vi "2025_day7.vi"() -> ()   [LabVIEW 2025]
uses:
  <userlib>/_OpenG.lib/string/string.llb/openg_string.lvlib
panel:
  out "Task 2":i64
  out "Task 1":i32
  in  "Switch":bool caption="Ex. Data  vs.  User Data"
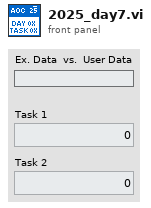
[diagram p1: front panel]
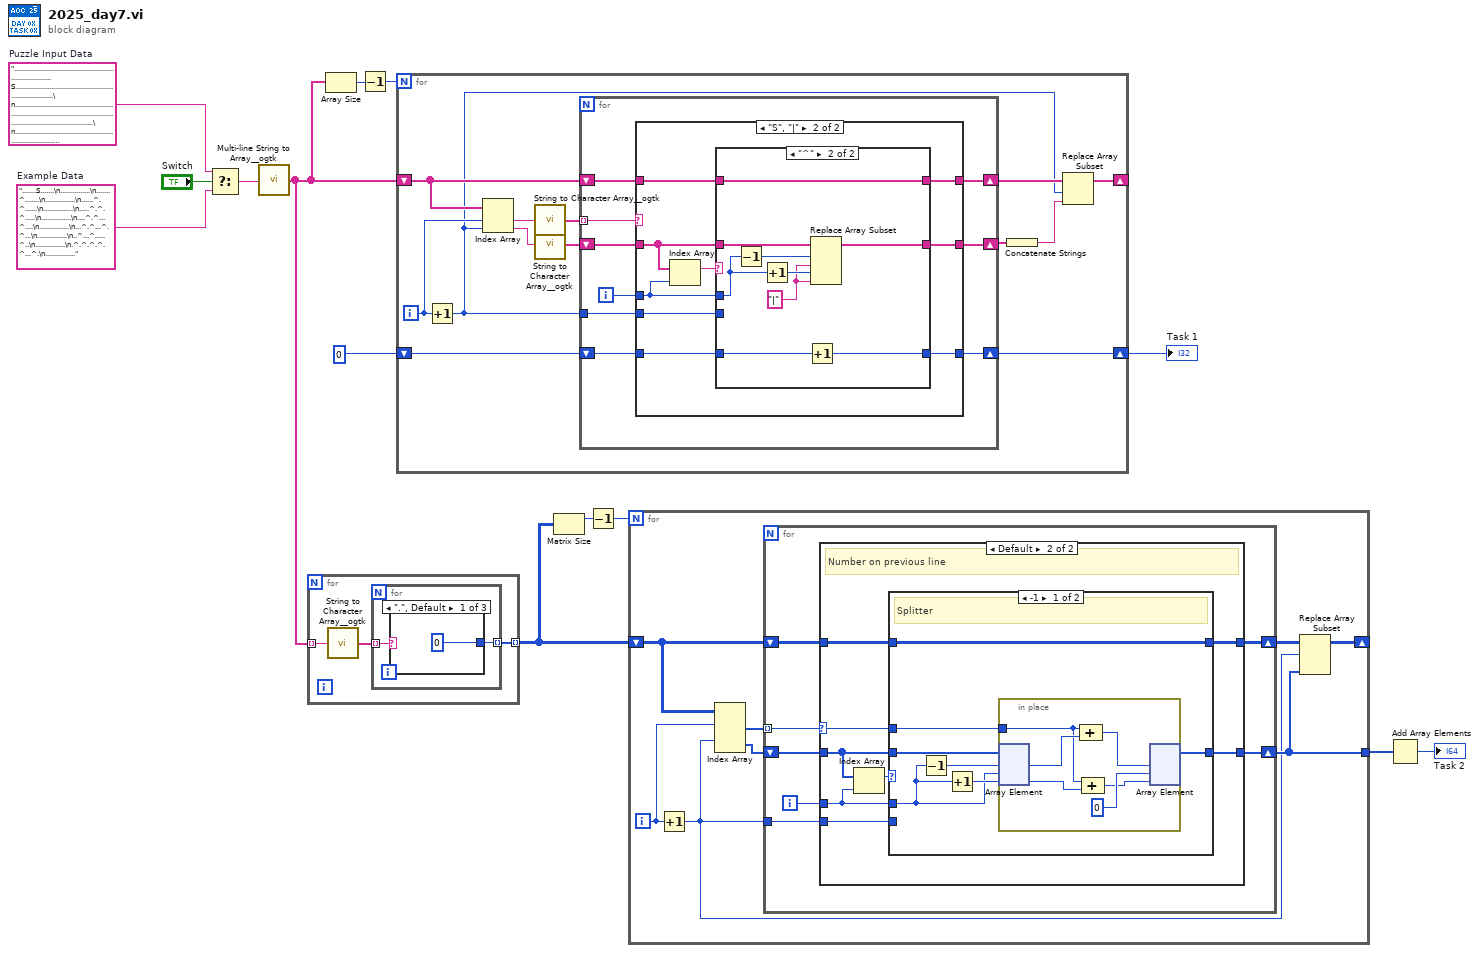
[diagram p0: block diagram]
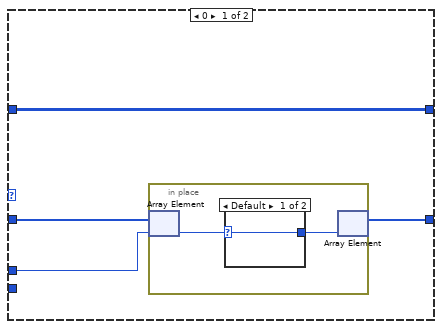
[diagram p2: hidden frame]
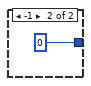
[diagram p3: hidden frame]
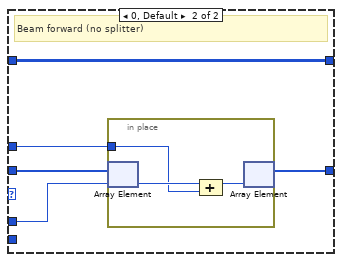
[diagram p4: hidden frame]
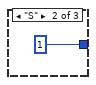
[diagram p5: hidden frame]
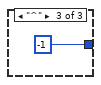
[diagram p6: hidden frame]
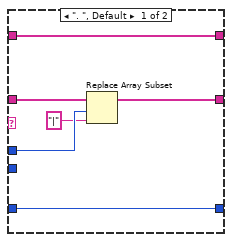
[diagram p8: hidden frame]
diagram:
  w12 = "......................................................................S......................................................................\n.............................................................................................................................................\n......................................................................^......................................................................\n.............................................................................................................................................\n.....................................................................^.^.....................................................................\n.............................................................................................................................................\n....................................................................^.^.^....................................................................\n.............................................................................................................................................\n...................................................................^.^.^.^...................................................................\n.............................................................................................................................................\n..................................................................^.^.^...^..................................................................\n.............................................................................................................................................\n.................................................................^.^.^.^.^.^.................................................................\n.............................................................................................................................................\n................................................................^.....^.^.^.^................................................................\n.............................................................................................................................................\n...............................................................^...^.^...^.^.^...............................................................\n.............................................................................................................................................\n..............................................................^.^.^.^...^.^.^.^..............................................................\n.............................................................................................................................................\n.............................................................^.^.^.^.^.^.^.^.^.^.............................................................\n.............................................................................................................................................\n............................................................^.^.^.^.^.^...^.^...^............................................................\n.............................................................................................................................................\n...........................................................^.^.^.^...^.^.^...^.^.^...........................................................\n.............................................................................................................................................\n..........................................................^.^.^...^.^.^.....^.^.^.^..........................................................\n.............................................................................................................................................\n.........................................................^.^...^...^.^.^.^...^.....^.........................................................\n.............................................................................................................................................\n........................................................^.....^.^.^...^.^.^.^.^.^.^.^........................................................\n.............................................................................................................................................\n.......................................................^.^...^.....^.......^.^.^.^...^.......................................................\n.............................................................................................................................................\n......................................................^.....^...^.^.^.^...^...^.^...^.^......................................................\n.............................................................................................................................................\n.....................................................^.^.^.^.^.^.^.^.^.....^.^.^.^...^.^.....................................................\n.............................................................................................................................................\n....................................................^.^.^.^...^.^...^.^.^...^...^.^.^.^.^....................................................\n.............................................................................................................................................\n...................................................^.....^.^.....^.^.^.^.....^.^.^.^.^.^.^...................................................\n.............................................................................................................................................\n..................................................^.^.^.^.^.^.^.......^...^.^.^.^.^.^.^.^.^..................................................\n.............................................................................................................................................\n.................................................^.....^...^.^.^.^.^...^.^.^.^.^.......^.^.^.................................................\n.............................................................................................................................................\n................................................^.^.^.....^.^.^.^.^.^.^.^.^.^.^.....^...^.^.^................................................\n.............................................................................................................................................\n...............................................^.^...^.^...^...^.^...^.^...^.^.^.^.^.^...^.^.^...............................................\n.............................................................................................................................................\n..............................................^.^.^.^...^.^.^.........^.^.^...^.^...^.^...^.^.^..............................................\n.............................................................................................................................................\n.............................................^.....^.^.^...^.^.^.^...^.^.^.^.^.^.^.^.^...^.^.^.^.............................................\n.............................................................................................................................................\n............................................^...^.....^.^.....^...^.^...^.^.^...^.^.^.^.^.^.^...^............................................\n.............................................................................................................................................\n...........................................^...^.^...^.^.^.^...^.^.......^.......^.^...^.^...^...^...........................................\n.............................................................................................................................................\n..........................................^.^.^.^.^.^.^.....^...^.^...^.^...^...^.....^...^...^...^..........................................\n.............................................................................................................................................\n.........................................^.^.^...^...^.^.....^.^...^.^.^...^...^.....^.^.^.^.....^.^.........................................\n.............................................................................................................................................\n........................................^.^...^...^.^.^...^.^...^.^...^.^.....^.^.^.^.^.^.....^.^...^........................................\n.............................................................................................................................................\n.......................................^.^.^.^.^.^.^.^.^.....^.^.^.^.^.^.^.^.^.^.^.^.^.^...^.^.^...^.^.......................................\n.............................................................................................................................................\n......................................^.^.^.^.^.^...^.^.^.^...^.^.^...^.^.^...^...^.^.^.^...^.^.^.^.^.^......................................\n.............................................................................................................................................\n.....................................^.^.^.^.^.^.^.........^.....^.^.....^.^.....^.^.^.^.^...^...^...^.^.....................................\n.............................................................................................................................................\n....................................^.^...^.........^.^.^.^.^.^...^.^.....^.^.....^...^.^...^.^...^...^.^....................................\n.............................................................................................................................................\n...................................^.^.^...^...^.^.^.^.^.^.^...^.^.^.^...^.^.^.^.....^.^.^.^.^...^...^.^.^...................................\n.............................................................................................................................................\n..................................^.....^.^.^.^.......^.....^.^.^.^.^.....^...^.^.^.....^.^.....^.^...^...^..................................\n.............................................................................................................................................\n.................................^...^.^.....^...^.^...^...^.^.....^...^.^.^.....^.^.......^.^.^.^.^.^...^.^.................................\n.............................................................................................................................................\n................................^.^.^.^.^.^...^.^.^.^.^.^...^...^.^.^.^...^.^...^.^.....^.^.^.....^.^...^.^.^................................\n.............................................................................................................................................\n...............................^.^.^.^.^.^.....^.^...^.^.^.^...^.^.^.^.^.^.^.^...^.^...^.^.^.^.^.......^.^.^.^...............................\n.............................................................................................................................................\n..............................^.^...^.^.......^...^...^.^...^.^.^.^.^...^.^.^.^.^.^.....^.^.^...^.......^...^.^..............................\n.............................................................................................................................................\n.............................^.^...^...^...^.^...^.^.^.^.....^.^.^.....^...^...^.......^...^.^.^.^.^.^.^.......^.............................\n.............................................................................................................................................\n............................^.^.^...^...^.^.^.^.^...^.^.^.^.^.^.^.^.^.^.^.^.^.^.......^.^.^.^.^.^.^.^.^.^.^.^.^.^............................\n.............................................................................................................................................\n...........................^.^...^.^.^.......^.^.....^.^.^...^.....^.^.^.....^.^.^.^.^.^.^.^...^.^.^.^.....^.^.^.^...........................\n.............................................................................................................................................\n..........................^.^.^.^.....^.^.....^.^.^.^.^.^.^...^.....^.^.^.^.^...^.^.^.^.^.....^.^...^.^...^...^.^.^..........................\n.............................................................................................................................................\n.........................^.^.^.^.^.^.^.^...^.^...^.^...^.^.^.......^.^.^.^.^.^.^.^.^...^.^.....^.^.^.^.^.^.^.^.....^.........................\n.............................................................................................................................................\n........................^.^.^.^.^...^.^.^.^.^.^.^...^.^...^.^.....^.^.^.^.^.^.^.^.....^.....^...^.^.......^.^.^.^.^.^........................\n.............................................................................................................................................\n.......................^...^.......^.......^.^...^.^.^.^...^.^.....^.^.^...^.^.^...^...^.^...^.^.^.^...^.^...^.^.^.^.^.......................\n.............................................................................................................................................\n......................^.^.^.^.....^...^.^.^...^.^.^...^.^.^.^.^.^.^...^...^.^.^.^.^.^...^.^.^...^...^.^.^.^.^...^.^.^.^......................\n.............................................................................................................................................\n.....................^.^.^.^.^.^...^.^.^...^.^.^...^...^.^.^.^.^.^...^...^.^.^.^...^...^...^...^.^.^.^...^.^.^.....^.^.^.....................\n.............................................................................................................................................\n....................^.^.^.^...^.......^...^.^...^...^.^.^.^...^.^.^.^.^.^.^.^.^...^...^.^.^.^.^.^.^.^.^.^.....^.^.^.^.^.^....................\n.............................................................................................................................................\n...................^.^.^...^.^.....^.^.^.^...^.^.^.^.^.^.....^.....^.......^.....^...^.....^...^.^...^.......^.^...^.^.^.^...................\n.............................................................................................................................................\n..................^.^.^...^.^...^.^.^.^...^.^.^...^.^.^...^.^.^.^.^.^...^.^...^.^.^...^.^.^.^.^.^.^.^.......^.....^.^.^...^..................\n.............................................................................................................................................\n.................^...^.^...^...^...^.^.^.^.^.^.^.^.^.^.^.^.......^.^.^...^.^.^.^.^...^.^.^...^.^.^.^.^...^...^.^...^.......^.................\n.............................................................................................................................................\n................^.^.^.^...^...^.^...^.^.^...^.^...^...^.^.^...^.^.^.^...^.....^.^.^...^.^...^.^.^.^...^.^.^...^.^.....^...^.^................\n.............................................................................................................................................\n...............^.^.^.......^.^.^.^.^...^...^.^...^.^...^.^.^.^.^...^.^.^.^.^.^.^.^.^...^.^.^...^...^...^...^.^...^.^.^.^.^.^.^...............\n.............................................................................................................................................\n..............^.^.^.^.^...^.^.^.....^.^...^.^.^.^.^.^.^.^.^.^.^...^.^.^...^.^.^.^.^...^...^.^.^.....^.^.^.....^...^.^.^...^.^.^..............\n.............................................................................................................................................\n.............^...^.....^.^...^.^...^.^...^.^.^.^.^.......^.^.^.^.^...^.^.^...^.^.^.....^.^...^.^.^.^.....^.^.^.^.^...^.^.^.^.^.^.............\n.............................................................................................................................................\n............^.^...^.......^...^.^.^.^.^.^.^...^.^.^.^.^.^...^...^.^.^.^.....^...^...^...^.^.^.^.^...^.^.^...^.^...^.^.^.^.^...^.^............\n.............................................................................................................................................\n...........^.....^.^.^.^...^.^.^...^...^...^.^.^.......^.....^.^.^.^...^.^.^...^...^.^.^...^...^.....^.^.^.^.^...^...^.^.^.^.^.^.^...........\n.............................................................................................................................................\n..........^.....^.^.^.^...^.^.^...^.^...^.....^.^...^.^.^.^.^.^.^.^.^.^.^.^.^.^.^.^.^.^...^...^.^.^.^.^...^.^.^.^.^.^.^.^...^.^.^.^..........\n.............................................................................................................................................\n.........^.^.^.^.^.^...^.^.^...^.^.^...^.....^...^.^.^.........^.^...^.^.....^.^.^.^.^.^.^.^.......^.^.^.^.^.^.......^.^.^.^.^...^.^.........\n.............................................................................................................................................\n........^.....^.^...^.^.^...^.^...^.^.^.^...^...^.^...^.^.^...^.^.....^.^.^...^.^...^.^.^.^.^.^.^.^.^.^.^.^.^.^.^.^.^...^...^.^.^...^........\n.............................................................................................................................................\n.......^.^...^.^.^.^.^...^.^.^.^.....^.^...^.^.^.^.^.^...^.^...^.^.^.^.^.^...^.^.^.^.^.......^.^.^.^...^...^.^.^.^.^.^.^.^.^...^...^.^.......\n.............................................................................................................................................\n......^...^.^.^.^...^.^.^.^.^...^.......^.^...^.^.....^.......^.^.......^...^.^.^...^.....^.^...^.^.^.^.....^.^...^.....^.^.^.^.^.^.^.^......\n.............................................................................................................................................\n.....^.^.....^.^.^.^.^.^.^.^.^.^.^.^.^...^.^.^.^.^.^...^...^.^.^.^...^.^.^...^.....^.^.^.^.^...^.^.^.^.^.....^.^.^.^.....^...^.^.^.^.^.^.....\n.............................................................................................................................................\n....^.......^.....^.^...^...^.^.^.^...^.........^.^...........^.^.^.^...^.^.^...^.^.^.^...^.^.^.^...^.^.^...^.^.^.^.^.^.....^.^.^...^.^.^....\n.............................................................................................................................................\n...^...^...^.^.^.^.^...^...^.^.^.^.^...^.....^...^.^.^.^.^...^.^.^.^...^.^...^...^.....^.^.^.^.^.^.^.^.^.^.^.^...^.......^.^.^.^.^.^...^.^...\n.............................................................................................................................................\n..^.^.^...^.^.^.^.^.^.^.^.^.^.^.^.^.^.^.^...^.^.^.^.^...^...^.^...^.^.^.^.^.......^.....^...^.^.^.^.^.^.....^.......^.^...^.^...^...^...^.^..\n.............................................................................................................................................\n.^...^.^.^.^.^.^...^...^.^...^.^.^...^...^.^...^.^.^...^.^.^.^.^...^...^...^.......^.^...^.^...^.^...^.^...^...^.^.^...^.^.^...^.^.^...^.^.^.\n............................................................................................................................................."  # Puzzle Input Data
  w13 = ".......S.......\n...............\n.......^.......\n...............\n......^.^......\n...............\n.....^.^.^.....\n...............\n....^.^...^....\n...............\n...^.^...^.^...\n...............\n..^...^.....^..\n...............\n.^.^.^.^.^...^.\n..............."  # Example Data
  n1 = Select(t=w12, s="Switch", f=w13) -> (s? t:f=w11:string)
  n2 = call <userlib>:"Multi-line String to Array__ogtk.vi"("string"=w11) -> ("lines"=w6:string[])
  n3 = for {
    tunnel: w6 -> [w17] mode=indexing
    tunnel: [w15] -> w2 mode=indexing
    n4 = call <userlib>:"String to Character Array__ogtk.vi"("Input String"=w17) -> ("Character Array"=w16:string[])
    n5 = for {
      tunnel: w16 -> [w19] mode=indexing
      tunnel: [w18] -> w15 mode=indexing
      n6 = case shown="\".\", Default" w19 {
        tunnel: [i64 0 i64 1 i64 -1] -> w18
        frame ".", Default {
        }
        frame "S" {
        }
        frame "^" {
        }
      }
    }
  }
  n7 = Array Size(array=w6) -> (size(s)=w10:i32)
  n8 = Decrement(x=w10) -> (x-1=w9:i32)
  n9 = for {
    N: w9 -> [_]
    shift-right: [w26] -> _
    shift-left: w6 -> [w33]
    shift-right: [w28] -> w7
    shift-left: 0 -> [w27]
    i -> [w35]
    n10 = Increment(x=w35) -> (x+1=w23:i32)
    n11 = Index Array(array=w33, index #1=w35, index #2=w23) -> (element #1=w31:string, element #2=w34:string)
    n12 = call <userlib>:"String to Character Array__ogtk.vi"("Input String"=w31) -> ("Character Array"=w30:string[])
    n13 = call <userlib>:"String to Character Array__ogtk.vi"("Input String"=w34) -> ("Character Array"=w29:string[])
    n14 = for {
      shift-right: [w43] -> w32
      shift-left: w33 -> [w44]
      tunnel: w30 -> [w42] mode=indexing
      tunnel: w23 -> [w41]
      shift-right: [w38] -> w25
      shift-left: w29 -> [w39]
      shift-right: [w37] -> w28
      shift-left: w27 -> [w36]
      i -> [w40]
      n15 = case shown="\"S\", \"|\"" w42 {
        tunnel: w44 -> [w47 w55]
        tunnel: [w47 w56] -> w43
        tunnel: w39 -> [w46 w51]
        tunnel: w41 -> [_ w54]
        tunnel: w40 -> [_ w53]
        tunnel: [w46 w50] -> w38
        tunnel: [w45 w49] -> w37
        tunnel: w36 -> [w45 w48]
        frame ".", Default {
        }
        frame "S", "|" {
          n16 = Index Array(array=w51, index=w53) -> (element=w52:string)
          n17 = case shown="\"^\"" w52 {
            tunnel: [w61 w71] -> w56
            tunnel: w55 -> [w61 w71]
            tunnel: w54 -> [_ _]
            tunnel: w53 -> [w59 w67]
            tunnel: w51 -> [w62 w70]
            tunnel: [w60 w69] -> w50
            tunnel: [w57 w63] -> w49
            tunnel: w48 -> [w57 w64]
            frame ". ", Default {
              n18 = Replace Array Subset(array=w62, new element="|" ("new element/subarray"), index=w59) -> (w60:string[])
            }
            frame "^" {
              w65 = "|" ("new element/subarray")
              n19 = Decrement(x=w67) -> (x-1=w68:i32)
              n20 = Increment(x=w67) -> (x+1=w66:i32)
              n21 = Increment(x=w64) -> (x+1=w63:i32)
              n22 = Replace Array Subset(array=w70, new element #1=w65, index #1=w68, new element #2=w65, index #2=w66) -> (w69:string[])
            }
          }
        }
      }
    }
    n23 = Concatenate Strings(w25) -> (w24:string)
    n24 = Replace Array Subset(array=w32, new element=w24, index=w23) -> (w26:string[])
  }
  "Task 1" <- w7
  n25 = Matrix Size(0:w2) -> (1:w5:i32)  [unwired: 1 out]
  n26 = Decrement(x=w5) -> (x-1=w1:i32)
  n27 = for {
    N: w1 -> [_]
    shift-right: [w72] -> _
    shift-left: w2 -> [w78]
    tunnel: [w75] -> w4
    i -> [w79]
    n28 = Increment(x=w79) -> (x+1=w74:i32)
    n29 = Index Array(array=w78, index (row) #1=w79, index (row) #2=w74) -> (element #1=w73:i64[], element #2=w76:i64[])  [unwired: 2 in]
    n30 = for {
      shift-right: [w85] -> w77
      shift-left: w78 -> [w86]
      tunnel: w73 -> [w84] mode=indexing
      tunnel: w74 -> [w83]
      shift-right: [w80] -> w75
      shift-left: w76 -> [w81]
      i -> [w82]
      n31 = case shown="Default" w84 {
        selector: w84 -> [_ w95]
        tunnel: w86 -> [w90 w101]
        tunnel: [w90 w102] -> w85
        tunnel: w81 -> [w89 w97]
        tunnel: w83 -> [_ w100]
        tunnel: w82 -> [w87 w99]
        tunnel: [w88 w96] -> w80
        frame 0 {
          n32 = in-place {
            n33 = in-place-array #1(w89, w87) -> (w91:i64)
            n34 = case shown="Default" w91 {
              selector: w91 -> [w93 _]
              tunnel: [w93 i64 0 ("element")] -> w92
              frame Default {
              }
              frame -1 {
              }
            }
            n35 = in-place-array #1(w92) -> (w88:i64[])  [unwired: 1 out]
          }
        }
        frame Default {
          # "Number on previous line"
          n36 = Index Array(array=w97, index=w99) -> (element=w98:i64)
          n37 = case shown="-1" w98 {
            tunnel: [w109 w120] -> w102
            tunnel: w101 -> [w109 w120]
            tunnel: w100 -> [_ _]
            tunnel: w99 -> [w104 w117]
            tunnel: w97 -> [w108 w119]
            tunnel: [w107 w118] -> w96
            tunnel: w95 -> [w106 w116]
            frame -1 {
              # "Splitter"
              n38 = Decrement(x=w104) -> (x-1=w103:i32)
              n39 = Increment(x=w104) -> (x+1=w105:i32)
              n40 = in-place {
                in-place-border: w106 -> [w111]
                n41 = in-place-array #2(w108, w103, w104, w105) -> (w114:i64, w112:i64)  [unwired: 1 out]
                n42 = Compound Arithmetic op=ADD(w111, w114) -> (w113:i64)
                n43 = Compound Arithmetic op=ADD(w111, w112) -> (w110:i64)
                n44 = in-place-array #2(w113, i64 0 ("element"), w110) -> (w107:i64[])  [unwired: 3 out]
              }
            }
            frame 0, Default {
              # "Beam forward (no splitter)"
              n45 = in-place {
                in-place-border: w116 -> [w121]
                n46 = in-place-array #3(w119, w117) -> (w123:i64)
                n47 = Compound Arithmetic op=ADD(w123, w121) -> (w122:i64)
                n48 = in-place-array #3(w122) -> (w118:i64[])  [unwired: 1 out]
              }
            }
          }
        }
      }
    }
    n49 = Replace Array Subset(array=w77, new element=w75, index (row)=w74) -> (w72:i64[][])  [unwired: 1 in]
  }
  n50 = Add Array Elements(numeric array=w4) -> (sum=→"Task 2":i64)
